vi "UI remove ROI.vi"(7 "new ROI":T1={"beads track"=[], "Public"={"标题名"="", "文件路径"=path "", "通道名"=[], "ROI Descriptor out"={"Global Rectangle"=[], "Contours"=[]}, "cali end"=0.0, "array piezo"=[], "LUT_R"=[], " ROI descriptors "=[{"Global Rectangle"=[0, 0, 0, 0], "Contours"=[{"ID"=enum."External", "Type"=12, "Coordinates"=[0, 0, 0, 0, 0]}]}, {"Global Rectangle"=[26, 104, 126, 204], "Contours"=[{"ID"=enum."External", "Type"=12, "Coordinates"=[26, 104, 126, 204, 0]}]}, {"Global Rectangle"=[99, 99, 201, 201], "Contours"=[{"ID"=enum."External", "Type"=12, "Coordinates"=[200, 200, 100, 100, 0]}]}], "tdms ref"=refnum, "分子长度(um)"=0.0, "ROI num"=0, "ROI size num"=[], "测量模式"=enum."force clamp"}, "beads info"=[]} {"Public"."ROI descriptors"."Contours"."Type" items=["No Selection", "Point", "Line", "Rectangle", "Oval", "Polygon", "Freehand Region", "Annulus", "Unused2", "Unused3", "Broken Line", "Freehand Line", "Rotated Rectangle"]; "Public"."ROI Descriptor out"."Contours"."Type" items=["No Selection", "Point", "Line", "Rectangle", "Oval", "Polygon", "Freehand Region", "Annulus", "Unused2", "Unused3", "Broken Line", "Freehand Line", "Rotated Rectangle"]; "beads track"."centroid"."Y Centroid" format="%.2f"; "beads track"."centroid"."X Centroid" format="%.2f"; "beads track"."ROI Des out"."Contours"."Type" items=["No Selection", "Point", "Line", "Rectangle", "Oval", "Polygon", "Freehand Region", "Annulus", "Unused2", "Unused3", "Broken Line", "Freehand Line", "Rotated Rectangle"]}, 8 "error in (no error)":errorcluster caption="错误输入（无错误）", 11 "remove ROI ?":refnum<vi>) -> (0 "error out":errorcluster caption="错误输出", 2 "ROI info out":T1={"beads track"=[], "Public"={"标题名"="", "文件路径"=path "", "通道名"=[], "ROI Descriptor out"={"Global Rectangle"=[], "Contours"=[]}, "cali end"=0.0, "array piezo"=[], "LUT_R"=[], " ROI descriptors "=[{"Global Rectangle"=[0, 0, 0, 0], "Contours"=[{"ID"=enum."External", "Type"=12, "Coordinates"=[0, 0, 0, 0, 0]}]}, {"Global Rectangle"=[26, 104, 126, 204], "Contours"=[{"ID"=enum."External", "Type"=12, "Coordinates"=[26, 104, 126, 204, 0]}]}, {"Global Rectangle"=[99, 99, 201, 201], "Contours"=[{"ID"=enum."External", "Type"=12, "Coordinates"=[200, 200, 100, 100, 0]}]}], "tdms ref"=refnum, "分子长度(um)"=0.0, "ROI num"=0, "ROI size num"=[], "测量模式"=enum."force clamp"}, "beads info"=[]} {"Public"."ROI descriptors"."Contours"."Type" items=["No Selection", "Point", "Line", "Rectangle", "Oval", "Polygon", "Freehand Region", "Annulus", "Unused2", "Unused3", "Broken Line", "Freehand Line", "Rotated Rectangle"]; "Public"."ROI Descriptor out"."Contours"."Type" items=["No Selection", "Point", "Line", "Rectangle", "Oval", "Polygon", "Freehand Region", "Annulus", "Unused2", "Unused3", "Broken Line", "Freehand Line", "Rotated Rectangle"]; "beads track"."centroid"."Y Centroid" format="%.2f"; "beads track"."centroid"."X Centroid" format="%.2f"; "beads track"."ROI Des out"."Contours"."Type" items=["No Selection", "Point", "Line", "Rectangle", "Oval", "Polygon", "Freehand Region", "Annulus", "Unused2", "Unused3", "Broken Line", "Freehand Line", "Rotated Rectangle"]})   [LabVIEW 2017]
doc: "本VI 用于删除指定编号的ROI ，要求即便在高度读写的情况下也要能正确删除，因此本VI十分特殊，放在数据分析循环的末尾，确保每次删除的过程中下一次读取还没有开始，写入则已经结束，以保证删除操作的有效性。"
uses:
  vision test/ROI info.ctl
  control/Bead track.ctl
  control/beads public.ctl
  control/record mode.ctl
  control/bead info.ctl
  <vilib>/vision/Image Controls.llb/IMAQ Image.ctl
  control/Bead info action.ctl
panel:
  out "rem ROI":bool
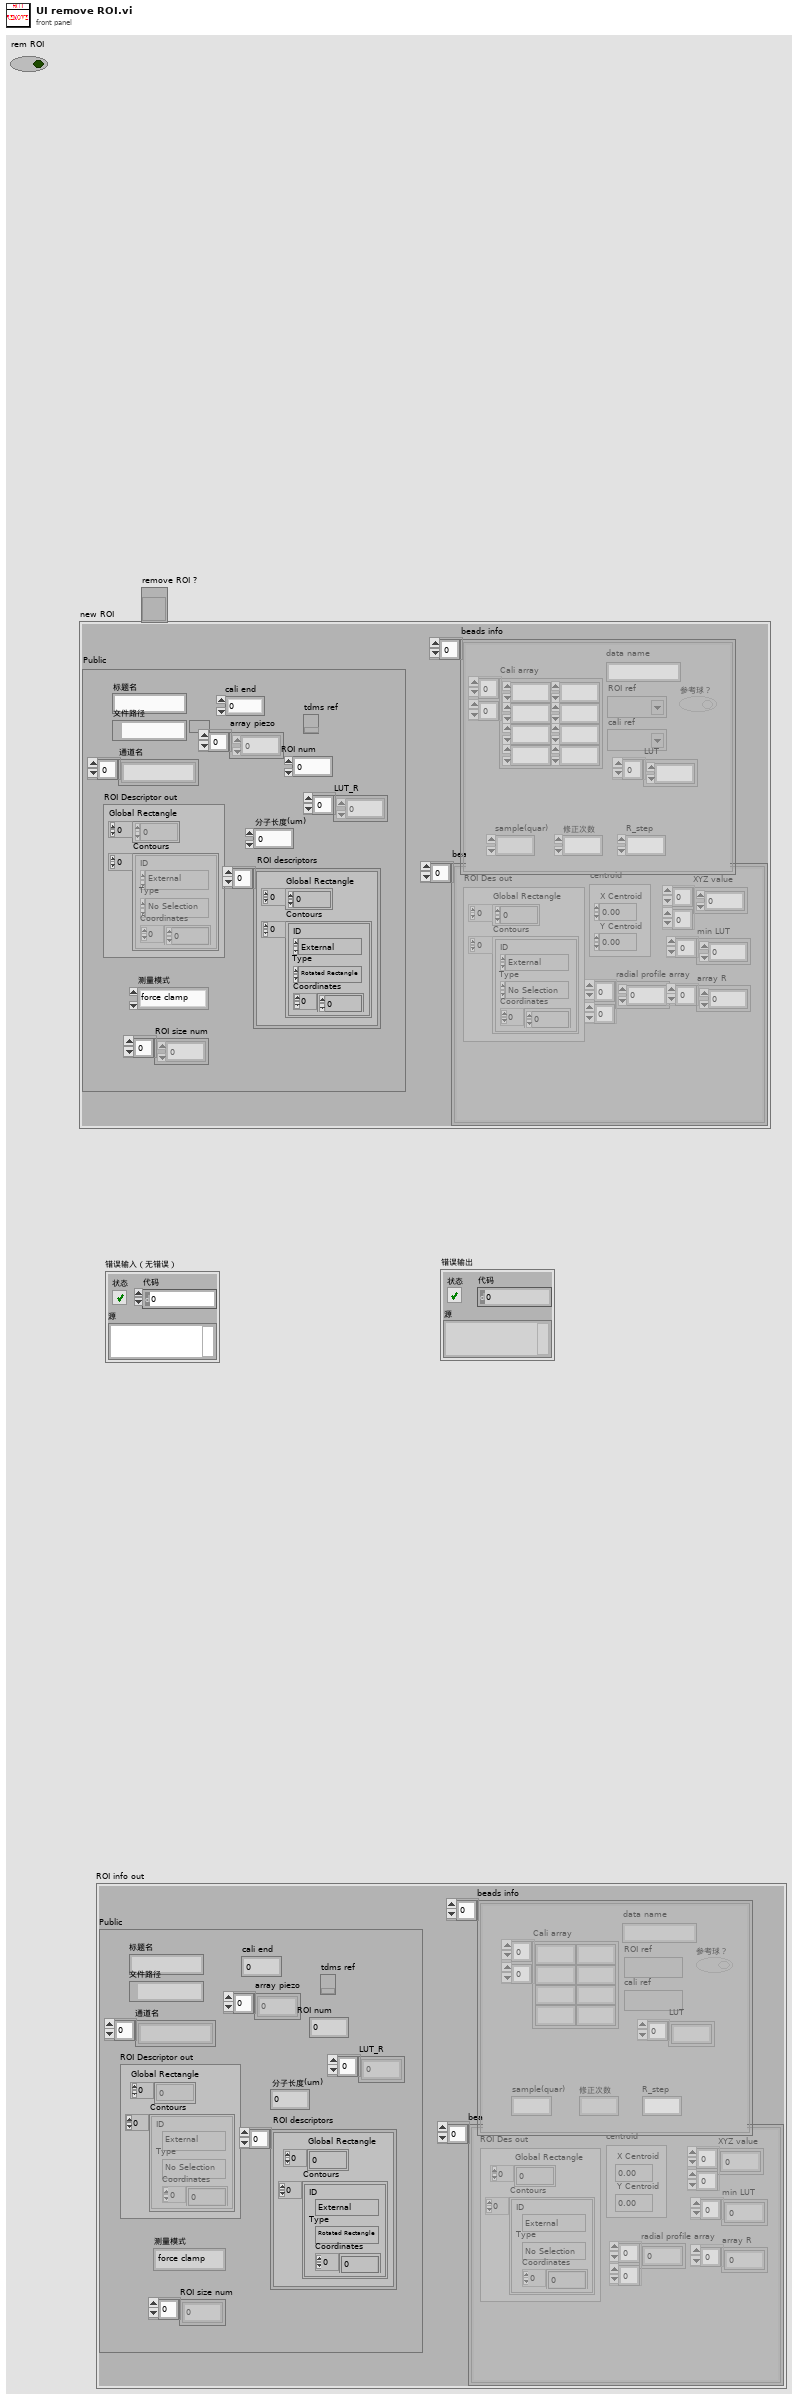
[diagram p1: front panel]
types:
  T1 = typedef "ROI info.ctl" = cluster{"beads track":T2[], "Public":T4, "beads info":T6[]}
  T2 = typedef "Bead track.ctl" = cluster{"XYZ value":dbl[][], "radial profile array":dbl[][], "min LUT":dbl[], "ROI Des out":T3, "array R":dbl[], "centroid":cluster{"X Centroid":sgl, "Y Centroid":sgl}}
  T3 = typedef "ROI Descriptor" = cluster{"Global Rectangle":i32[], "Contours":cluster{"ID":enum32{"External", "Internal"}, "Type":u32, "Coordinates":i32[]}[]}
  T4 = typedef "beads public.ctl" = cluster{"标题名":string, "文件路径":path, "通道名":string[], "ROI Descriptor out":T3, "cali end":dbl, "array piezo":dbl[], "LUT_R":dbl[], " ROI descriptors ":T3[], "tdms ref":refnum<k34>, "分子长度(um)":dbl, "ROI num":i32, "ROI size num":i32[], "测量模式":T5}
  T5 = typedef "record mode.ctl" = enum16{"force ramp", "force clamp", "user-defined", "force-mixed"}
  T6 = typedef "bead info.ctl" = cluster{"data name":string, "ROI ref":T7, "cali ref":T7, "参考球？":bool, "LUT":dbl[], "Cali array":dbl[][], "修正次数":i32, "R_step":dbl, "sample(quar)":i32}
  T7 = typedef "IMAQ Image.ctl" = refnum<image>
  T8 = typedef "Bead info action.ctl" = enum16{"read", "write track", "intial", "write info", "write all", "write public"}
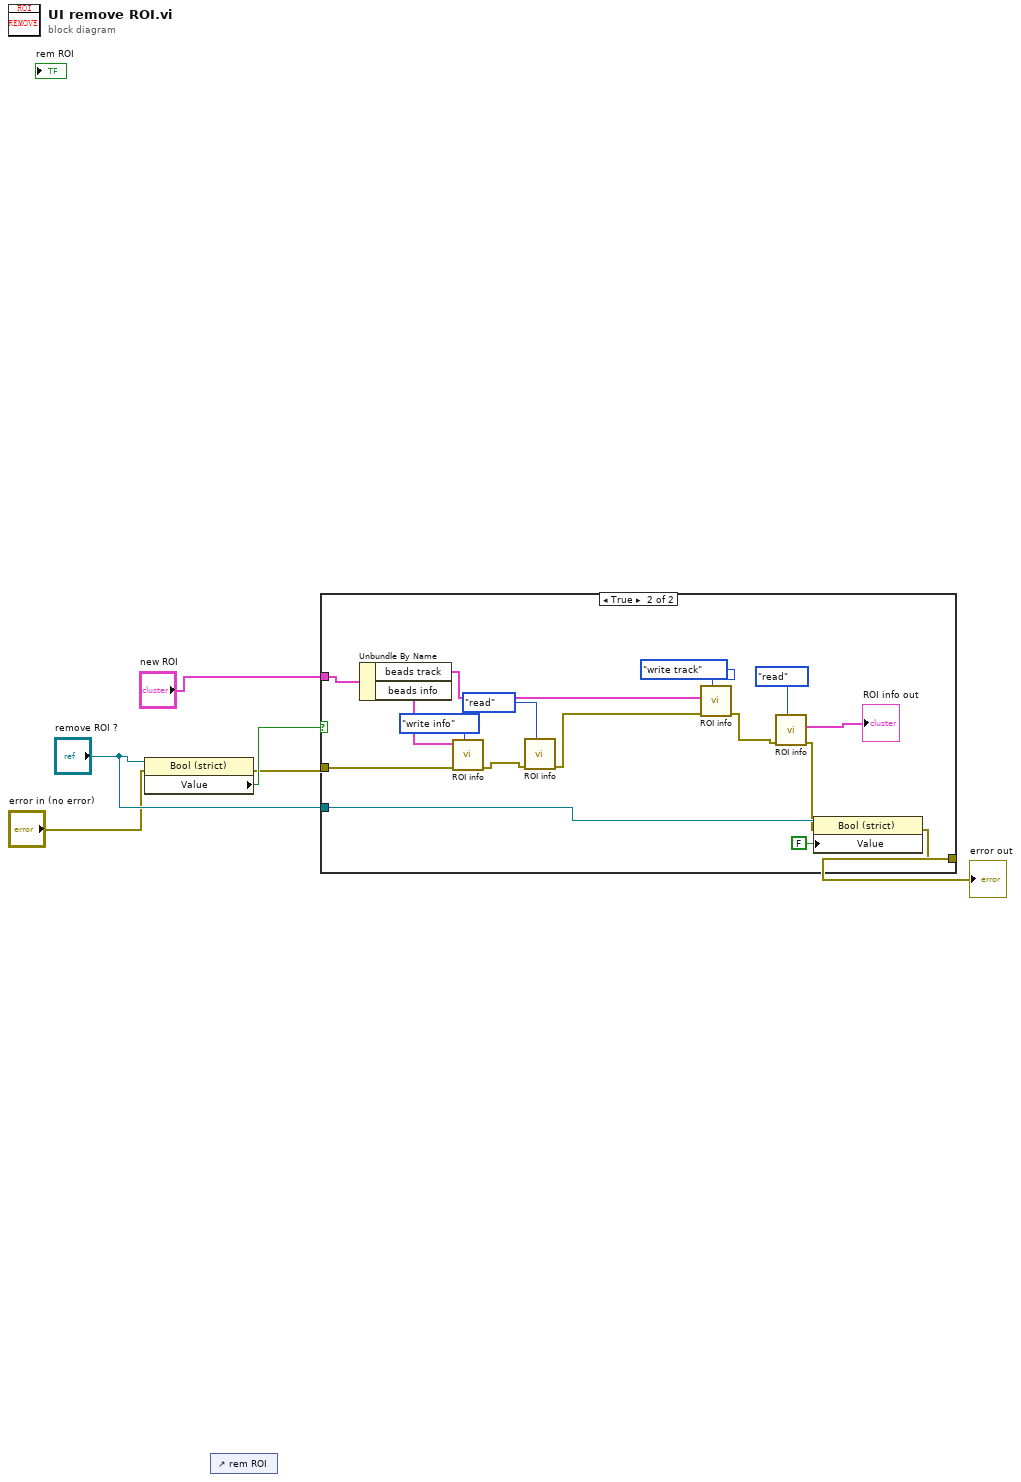
[diagram p0: block diagram]
diagram:
  n1 = property on="属性节点" class="Bool (strict)"(reference="remove ROI ?", error in="error in (no error)") -> (error out=w4:errorcluster, "Value"=w5:bool)  [unwired: 1 out]
  n2 = control-ref of="rem ROI"() -> ()  [unwired: 1 out]
  n3 = case shown="True" w5 {
    tunnel: "new ROI" -> [_ w23]
    tunnel: w4 -> [w7 w19]
    tunnel: "remove ROI ?" -> [_ w17]
    tunnel: [w7 w16] -> w1
    frame False {
    }
    frame True {
      n4 = Unbundle By Name(w23) -> ("beads track"=w20:T2[], "beads info"=w21:T6[])
      n5 = call "ROI info.vi"("action"=Bead_info_action."write info", "error in (no error)"=w19, "beads info"=w21) -> ("error out"=w14:errorcluster)  [unwired: 7 in, 1 out]
      n6 = call "ROI info.vi"("action"=Bead_info_action."read", "error in (no error)"=w14) -> ("error out"=w12:errorcluster)  [unwired: 8 in, 1 out]
      n7 = call "ROI info.vi"("action"=Bead_info_action."write track", "error in (no error)"=w12, "beads track"=w20) -> ("error out"=w11:errorcluster)  [unwired: 7 in, 1 out]
      n8 = call "ROI info.vi"("action"=Bead_info_action."read", "error in (no error)"=w11) -> ("error out"=w8:errorcluster, "ROI info out"=→"ROI info out":T1)  [unwired: 8 in]
      n9 = property on="属性节点" class="Bool (strict)"(reference=w17, error in=w8, "Value"=FALSE ("值")) -> (error out=w16:errorcluster)  [unwired: 1 out]
    }
  }
  "error out" <- w1
